vi "Normalize Coordinates.vi"(6 "Camera Distance\nfrom Ground (in)":dbl, 8 "Distance Method":u16(ring) items=["Default", "Center Calculations", "Hybrid"], 9 "Camera Type":T2, 10 "Targets":T5(array[cluster]), 11 "Image in":T6) -> (1 "Array":T1(array[cluster]), 2 "Found Targets":T3(array[cluster]) {"Normalized Rect"."Numeric 5" format="%#_2g"; "Normalized Rect"."Numeric 3" format="%#_2g"; "Normalized Rect"."Numeric 2" format="%#_2g"; "Normalized Rect"."Numeric" format="%#_2g"}, 3 "Sorted Scores":T4(array[cluster]) {"Moment Factor" format="%#_3g"; "L" format="%#_3g"; "Area to CH" format="%#_3g"; "X" format="%#_3g"; "Y" format="%#_3g"})   [LabVIEW 2015]
doc: "Normalize the rectangle and center so that they range from -1 to 1, left to right and bottom to top. This helps with producing joystick coordinates for driving the robot and makes the code better at handling resolution changes of the camera."
uses:
  <vilib>/vision/Image Controls.llb/IMAQ Image.ctl
  Camera Types.ctl
panel:
  # "Aspect Ratio"
  # "Density Profile"
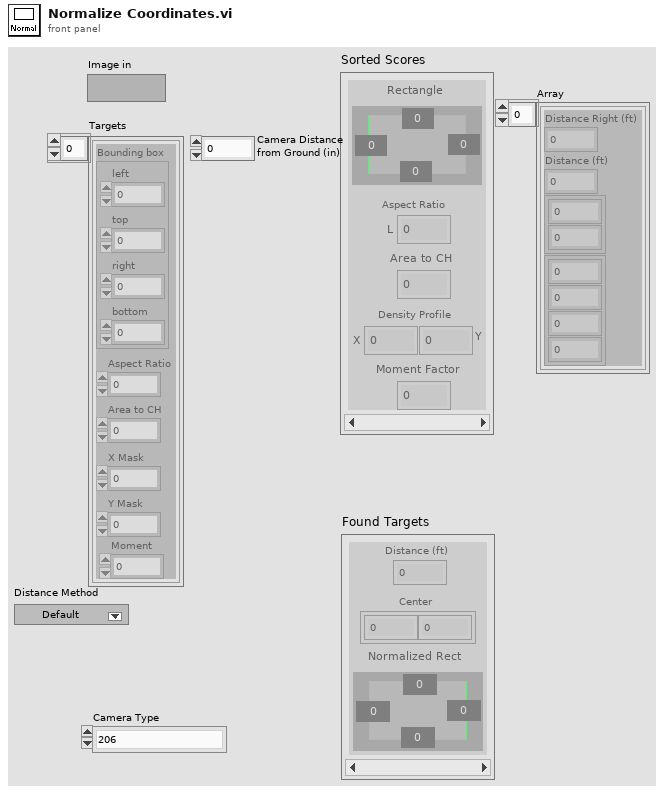
[diagram p1: front panel]
types:
  T1 = cluster{"Distance Right (ft)":dbl, "Distance (ft)":dbl, cluster{dbl, dbl}, cluster{dbl, dbl, dbl, dbl}}[]
  T2 = typedef "Camera Types.ctl" = enum16{"206", "1011", "1013", "MS HD3000 square", "MS HD3000 640x480"}
  T3 = cluster{"Distance (ft)":dbl, "Center":cluster{dbl, dbl}, "Normalized Rect":cluster{"Numeric":dbl, "Numeric 2":dbl, "Numeric 3":dbl, "Numeric 5":dbl}}[]
  T4 = cluster{"Rectangle":cluster{"Numeric":dbl, "Numeric 2":dbl, "Numeric 3":dbl, "Numeric 5":dbl}, "L":dbl, "Area to CH":dbl, "X":dbl, "Y":dbl, "Moment Factor":dbl}[]
  T5 = cluster{"Bounding box":cluster{"left":dbl, "top":dbl, "right":dbl, "bottom":dbl}, "Aspect Ratio":dbl, "Area to CH":dbl, "X Mask":dbl, "Y Mask":dbl, "Moment":dbl}[]
  T6 = typedef "IMAQ Image.ctl" = refnum<image>
  T7 = cluster{"left":dbl, "top":dbl, "right":dbl, "bottom":dbl}
  T8 = cluster{"X Resolution":i32, i32, "X Resolution":i32, i32}
  T9 = cluster{"Distance Right (ft)":dbl, "Distance Back (ft)":dbl, cluster{dbl, dbl}, cluster{dbl, dbl, dbl, dbl}}
  T10 = cluster{"Distance Back (ft)":dbl, cluster{dbl, dbl}, cluster{dbl, dbl, dbl, dbl}}
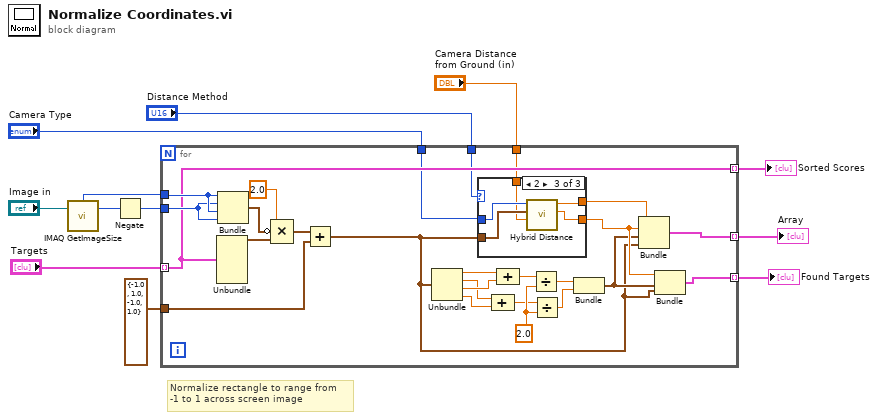
[diagram p0: block diagram]
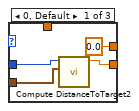
[diagram p2: hidden frame]
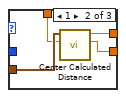
[diagram p3: hidden frame]
diagram:
  # "Normalize rectangle to range from\n-1 to 1 across screen image"
  n1 = call "IMAQ GetImageSize"("Image"="Image in") -> ("Y Resolution"=w10:i32, "X Resolution"=w11:i32)  [unwired: 3 in, 1 out]
  n2 = Negate(x=w10) -> (-x=w12:i32)
  n3 = for {
    tunnel: "Targets" -> [w22] mode=indexing
    tunnel: w12 -> [w37]
    tunnel: w11 -> [w38]
    tunnel: [w23] -> w4 mode=indexing
    tunnel: [w22] -> w5 mode=indexing
    tunnel: cluster{dbl, dbl, dbl, dbl} {-1.0, 1.0, -1.0, 1.0} ("y") -> [w21]
    tunnel: "Camera Type" -> [w20]
    tunnel: [w15] -> w3 mode=indexing
    tunnel: "Camera Distance\nfrom Ground (in)" -> [w14]
    tunnel: "Distance Method" -> [w13]
    w28 = 2.0
    n4 = Unbundle(w22) -> ("Bounding box"=w35:T7)  [unwired: 5 out]
    n5 = Bundle("X Resolution"=w38, w37, "X Resolution"=w38, w37) -> (w36:T8)  [unwired: 1 in]
    n6 = Compound Arithmetic op=MULTIPLY(2.0, invert w36, w35) -> (w34:cluster{dbl, dbl, dbl, dbl})
    n7 = Add(x=w34, y=w21) -> (x+y=w16:cluster{dbl, dbl, dbl, dbl})
    n8 = Unbundle(w16) -> (w32:dbl, w29:dbl, w31:dbl, w30:dbl)
    n9 = case shown="2" w13 {
      tunnel: [w42 w45 w47] -> w18
      tunnel: w20 -> [w41 _ w51]
      tunnel: w16 -> [w40 w46 w50]
      tunnel: [0.0 ("Distance Right (ft)") w44 w48] -> w19
      tunnel: w14 -> [_ w43 w49]
      frame 0, Default {
        n10 = call "Compute DistanceToTarget2.vi"("Normalized Rect"=w40, "Camera Type"=w41) -> ("Distance (ft)"=w42:dbl)  [unwired: 9 in]
      }
      frame 1 {
        n11 = call "Center Calculated Distance.vi"("Camera Distance\nfrom Ground (in)"=w43, "Normalized Rect"=w46) -> ("Distance (ft)"=w45:dbl, "Distance Right (ft)"=w44:dbl)  [unwired: 8 in]
      }
      frame 2 {
        n12 = call "Hybrid Distance.vi"("Camera Distance\nfrom Ground (in)"=w49, "Normalized Rect"=w50, "Camera Type"=w51) -> ("Distance Back (ft)"=w47:dbl, "Distance Right (ft)"=w48:dbl)  [unwired: 7 in]
      }
    }
    n13 = Compound Arithmetic op=ADD(w29, w30) -> (w26:dbl)
    n14 = Compound Arithmetic op=ADD(w32, w31) -> (w27:dbl)
    n15 = Divide(x=w27, y=w28) -> (x/y=w25:dbl)
    n16 = Divide(x=w26, y=w28) -> (x/y=w24:dbl)
    n17 = Bundle(w25, w24) -> (w17:cluster{dbl, dbl})  [unwired: 1 in]
    n18 = Bundle("Distance Right (ft)"=w19, "Distance Back (ft)"=w18, w17, w16) -> (w23:T9)  [unwired: 1 in]
    n19 = Bundle("Distance Back (ft)"=w18, w17, w16) -> (w15:T10)  [unwired: 1 in]
  }
  "Sorted Scores" <- w5
  "Found Targets" <- w3
  "Array" <- w4
